vi "main_v1.2.vi"() -> ()   [LabVIEW 2012]
uses:
  SensorSettingCtl.ctl
  SensorTypes.ctl
  states.ctl
  globalVariables.vi
  <vilib>/Analysis/NI_AALPro.lvlib
panel:
  out "mean current CAN - ANA new":dbl format="%#_5g"
  out "mean currents":dbl[](array[numeric]) format="%#_5g"
  out "min dt":dbl[](array[numeric])
  out "max dt":dbl[](array[numeric])
  out "dt":dbl[][](array[numeric])
  out "end-time / s":dbl[](array[numeric])
  out "start-time / s":dbl[](array[numeric])
  out "calculated sampling rates / s":dbl[](array[numeric]) format="%^#_5e"
  out "currents zoomed 2":cluster{dbl[], dbl[]}[](graph)
  out "zoomed currents":dbl[][](array[numeric])
  out "zoomed times":dbl[][](array[numeric])
  in  "autostart":bool=TRUE
  out "raw currents":dbl[][](array[numeric])
  in  "start-indices":i32[](array[numeric])
  in  "end-indices":i32[](array[numeric])
  out "raw times":dbl[][](array[numeric])
  in  "cancel button data analysis":bool
  out "meas. time / s":dbl format="%#.1f"
  in  "max. meas. time / s":dbl=10.0
  out "measuring":bool
  out "currents raw":cluster{dbl[], dbl[]}[](graph)
  out "currents zoomed":cluster{dbl[], dbl[]}[](graph)
  in  "size of buffer":i32=1000000
  in  "Path for measuring results":path=path "C:/Users/Induelec/Desktop/test_output"
  in  "Sensor types":T1[](array[typedef])=[enum."ITL 900 (Analogue)", enum."CAB 300-C SP3 (CAN)", enum."xyz TODO (PWM)", enum."xyz TODO (LIN)", enum."xyz TODO (Analogue)"]
  in  "Sensor-enabling":T2[](array[typedef])=[{"VISA resource name"="", "use sensor"=FALSE}, {"VISA resource name"="", "use sensor"=TRUE}, {"VISA resource name"="", "use sensor"=FALSE}, {"VISA resource name"="", "use sensor"=FALSE}, {"VISA resource name"="", "use sensor"=FALSE}]
  in  "cancel button":bool
  in  "start Button":bool
  out "Error Flag":bool
  # "Measurement of Current Sensors from LEM"
  # "ANA"
  # "CAN"
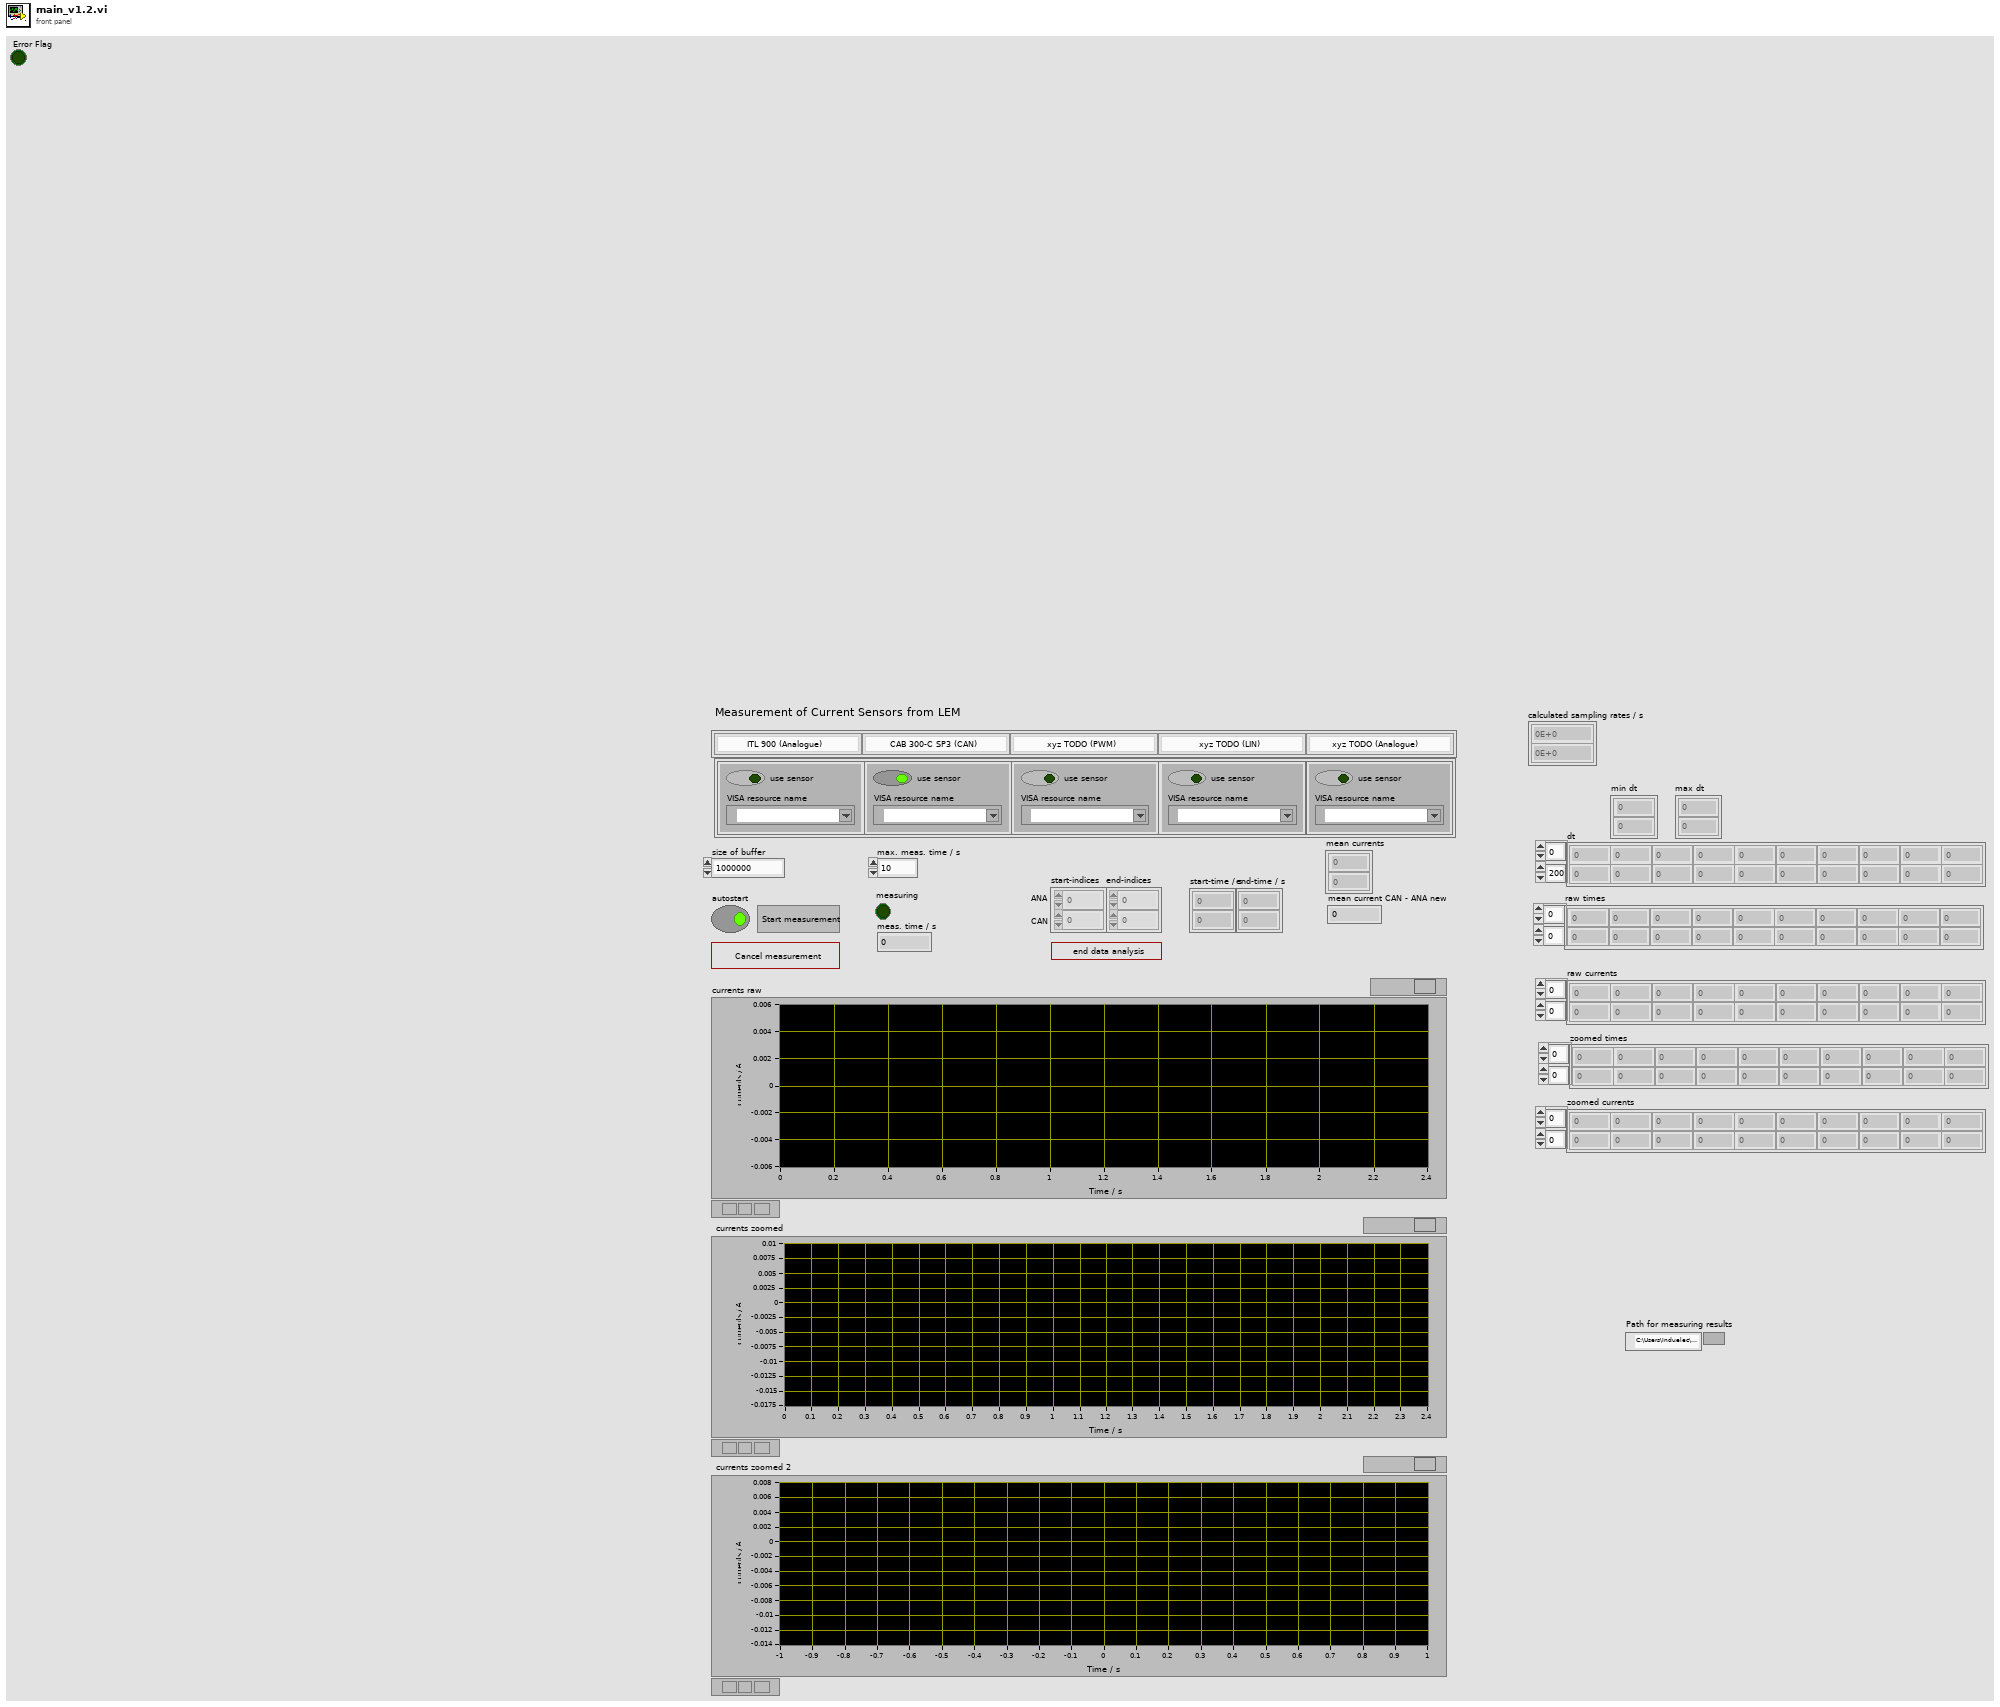
[diagram p1: front panel]
types:
  T1 = typedef "SensorTypes.ctl" = enum16{"ITL 900 (Analogue)", "CAB 300-C SP3 (CAN)", "xyz TODO (PWM)", "xyz TODO (LIN)", "xyz TODO (Analogue)"}
  T2 = typedef "SensorSettingCtl.ctl" = cluster{"VISA resource name":refnum<visa-resource-name>, "use sensor":bool}
  T3 = typedef "states.ctl" = enum16{"init", "wait for user confirm", "start sensors", "measure", "data preparation", "data analysis", "terminate"}
  T4 = typedef "Semaphore RefNum" = refnum<k1>
  T5 = typedef "TimeValue.ctl" = cluster{"Time of measurement":timestamp, "Current value":dbl}
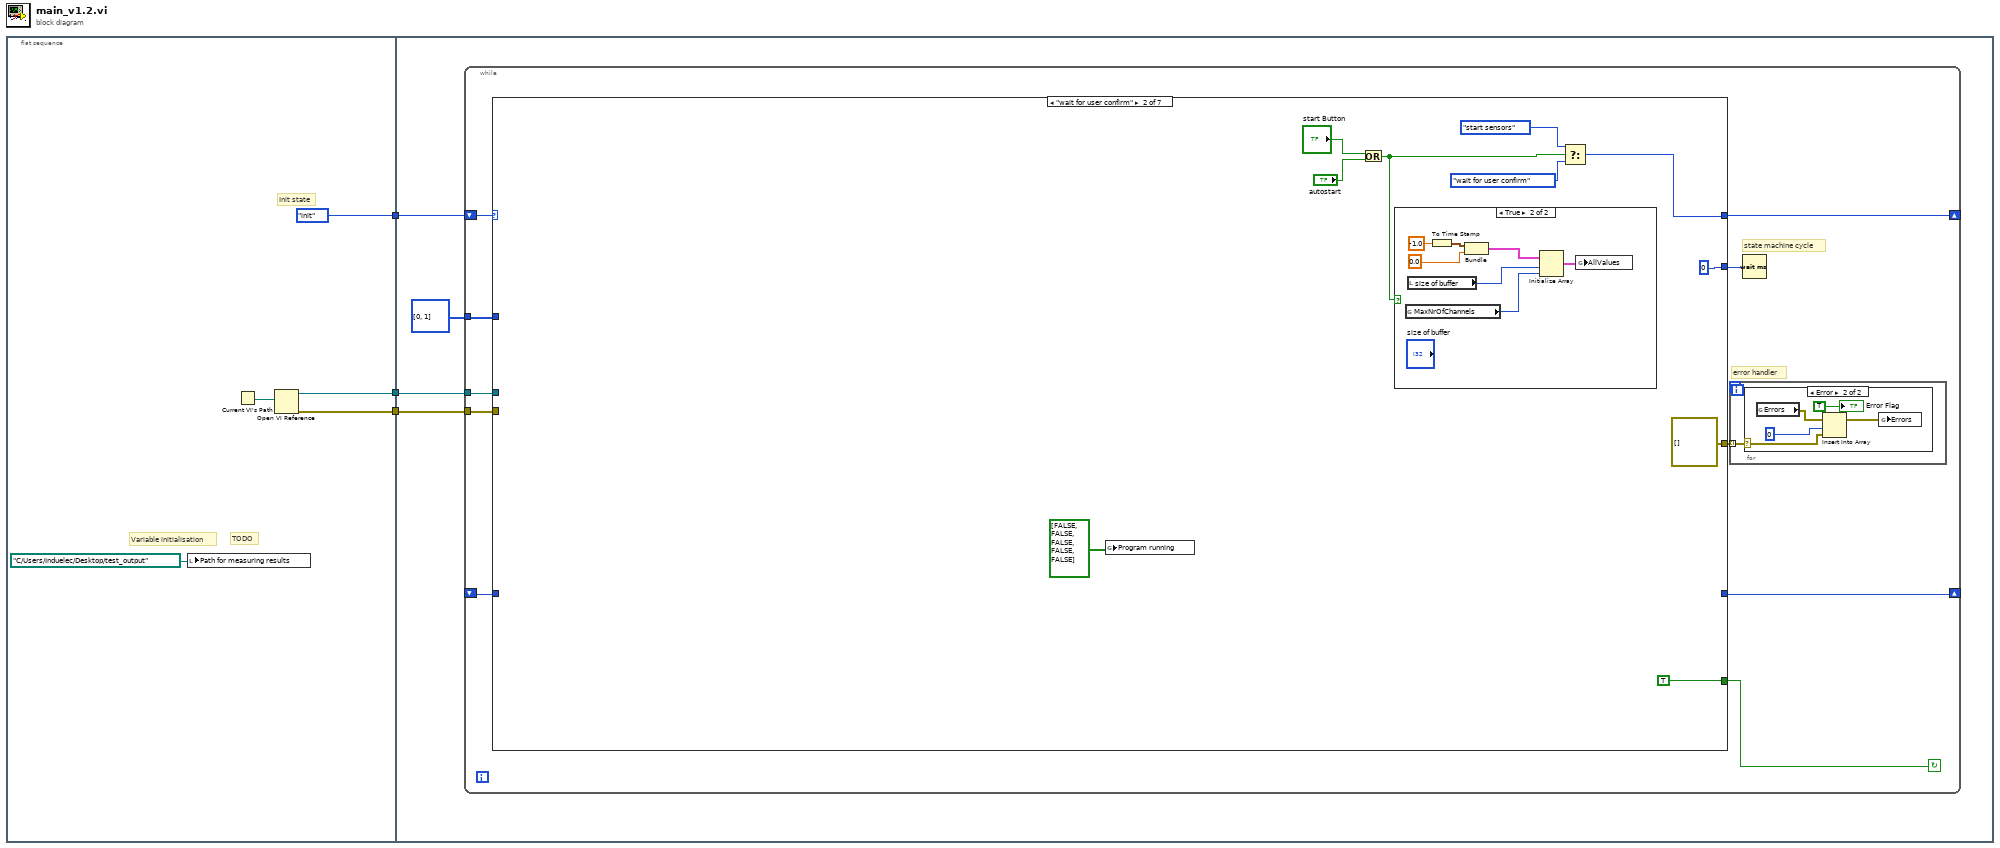
[diagram p0: block diagram]
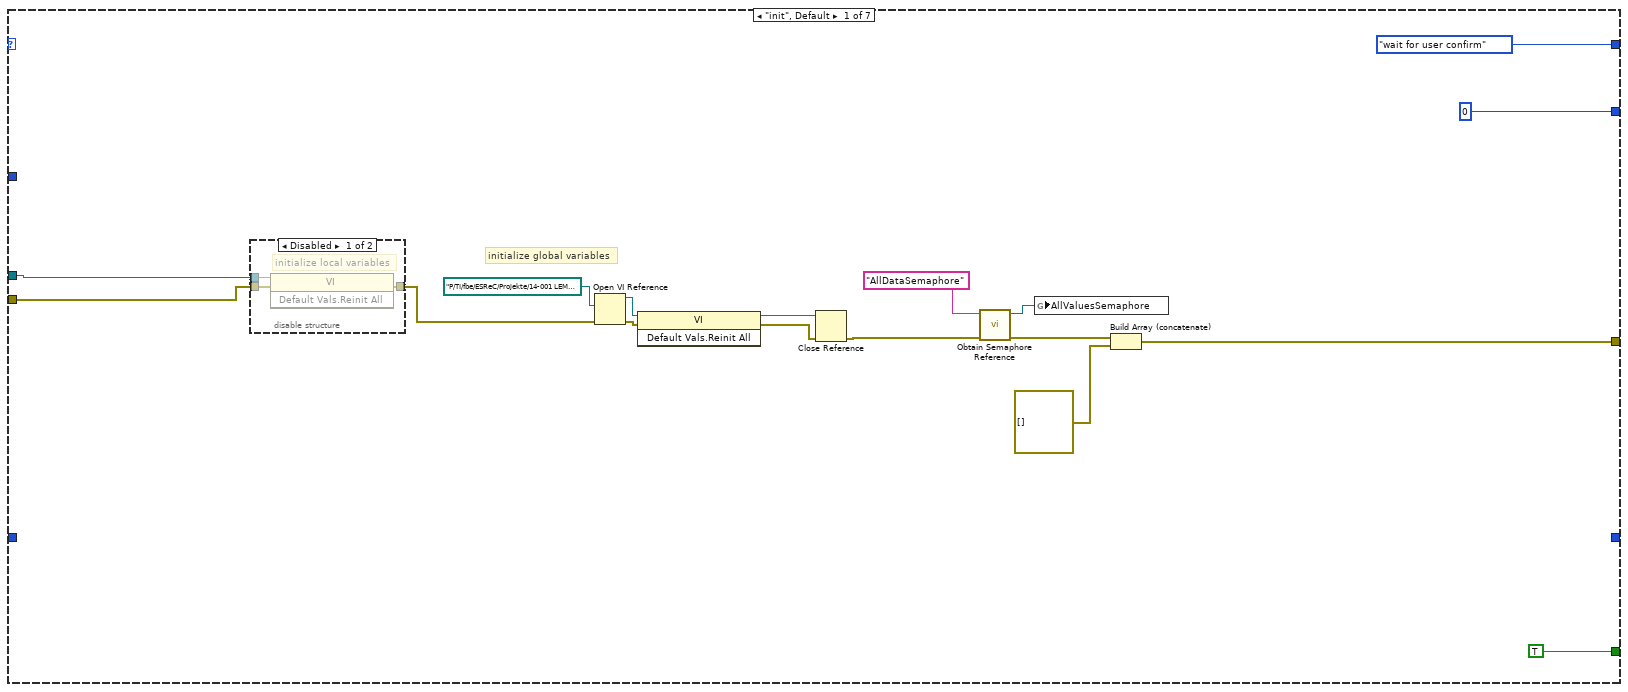
[diagram p3: hidden frame]
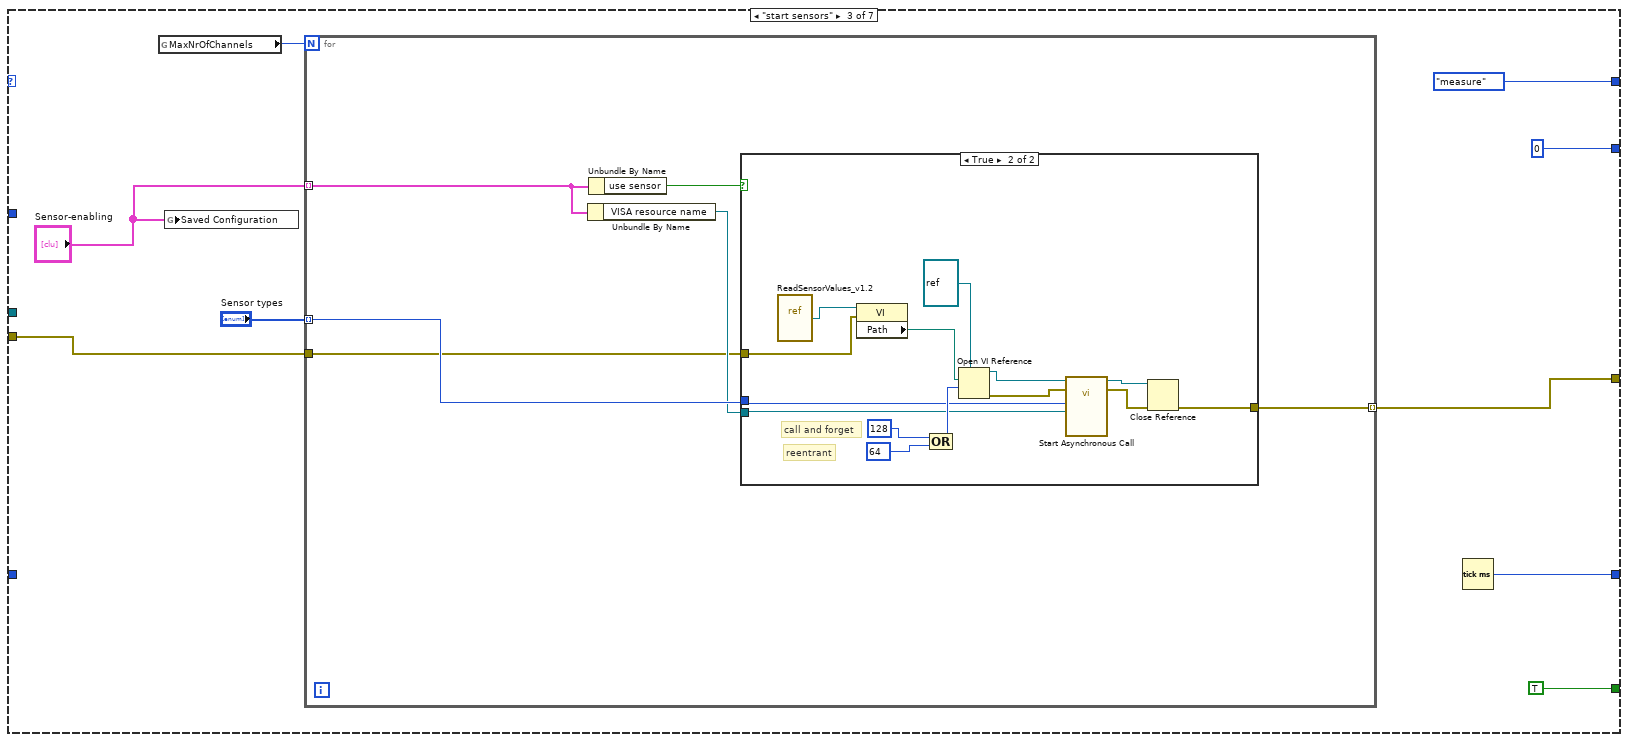
[diagram p6: hidden frame]
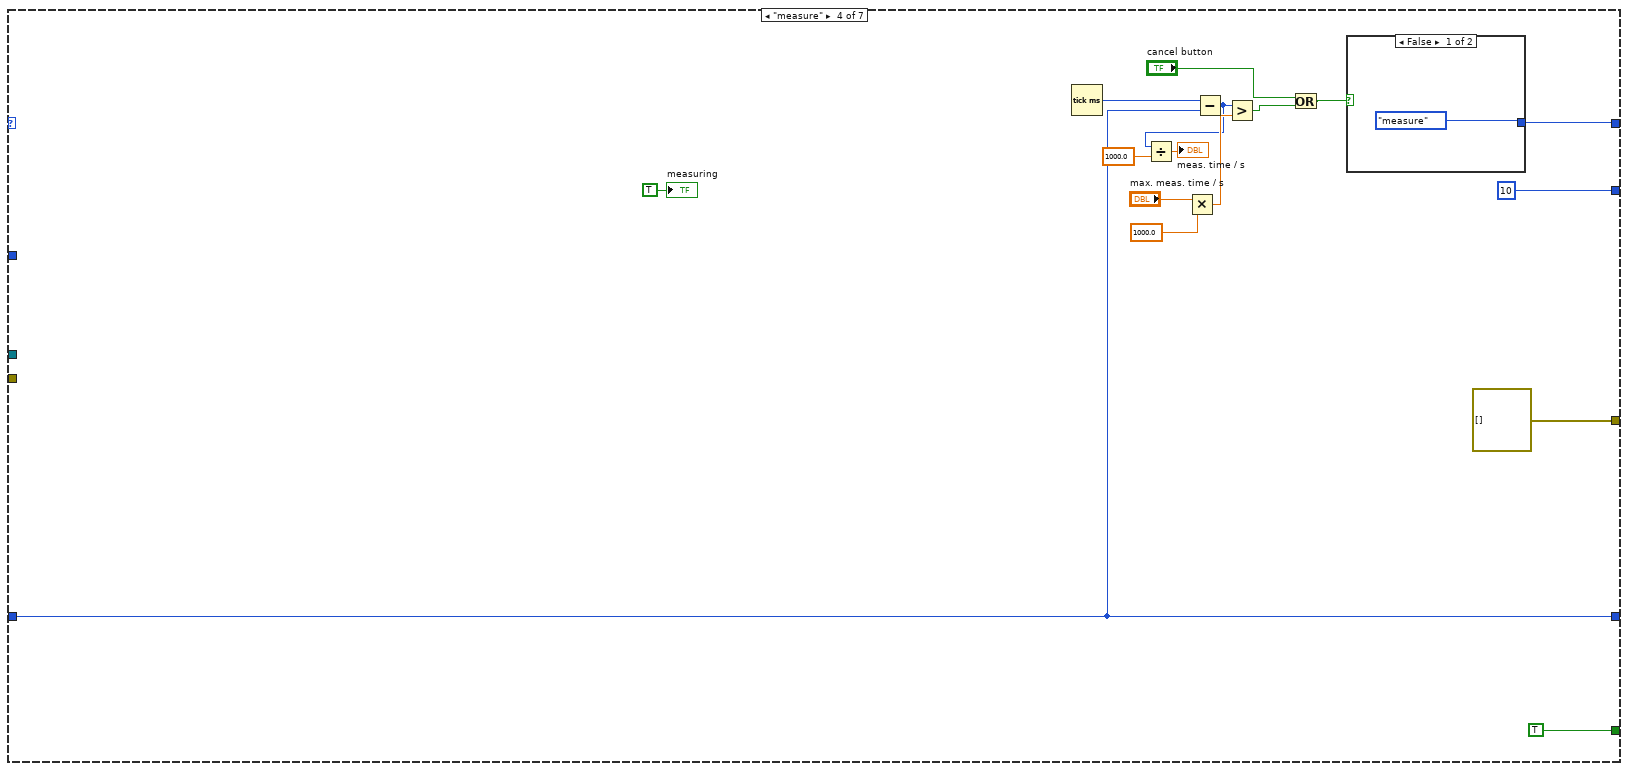
[diagram p8: hidden frame]
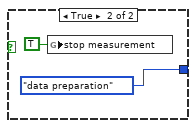
[diagram p9: hidden frame]
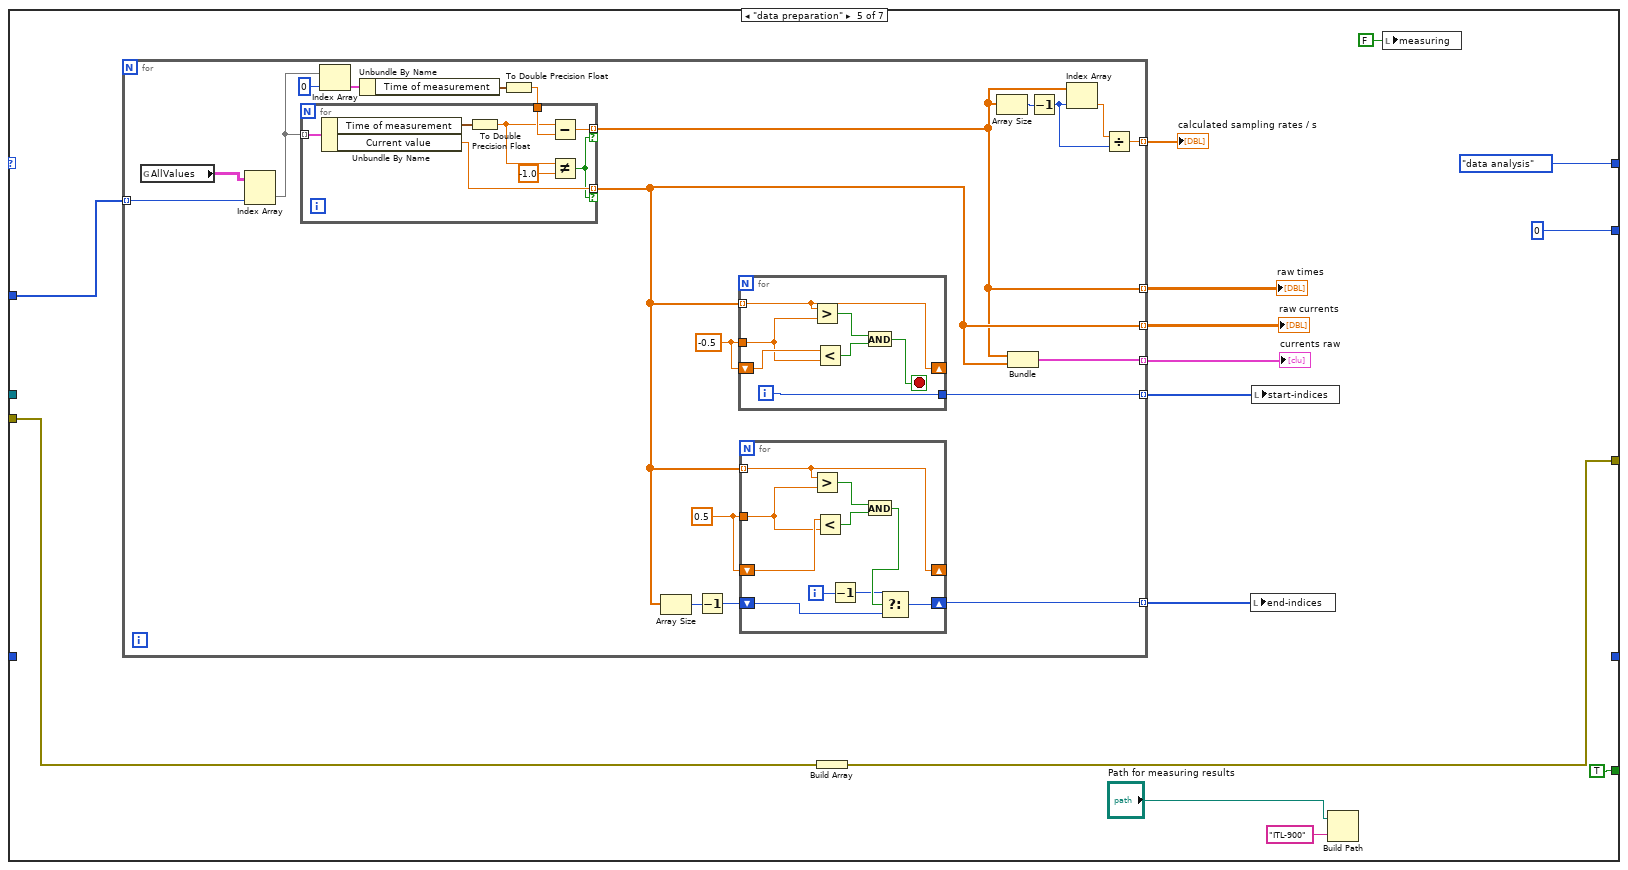
[diagram p10: hidden frame]
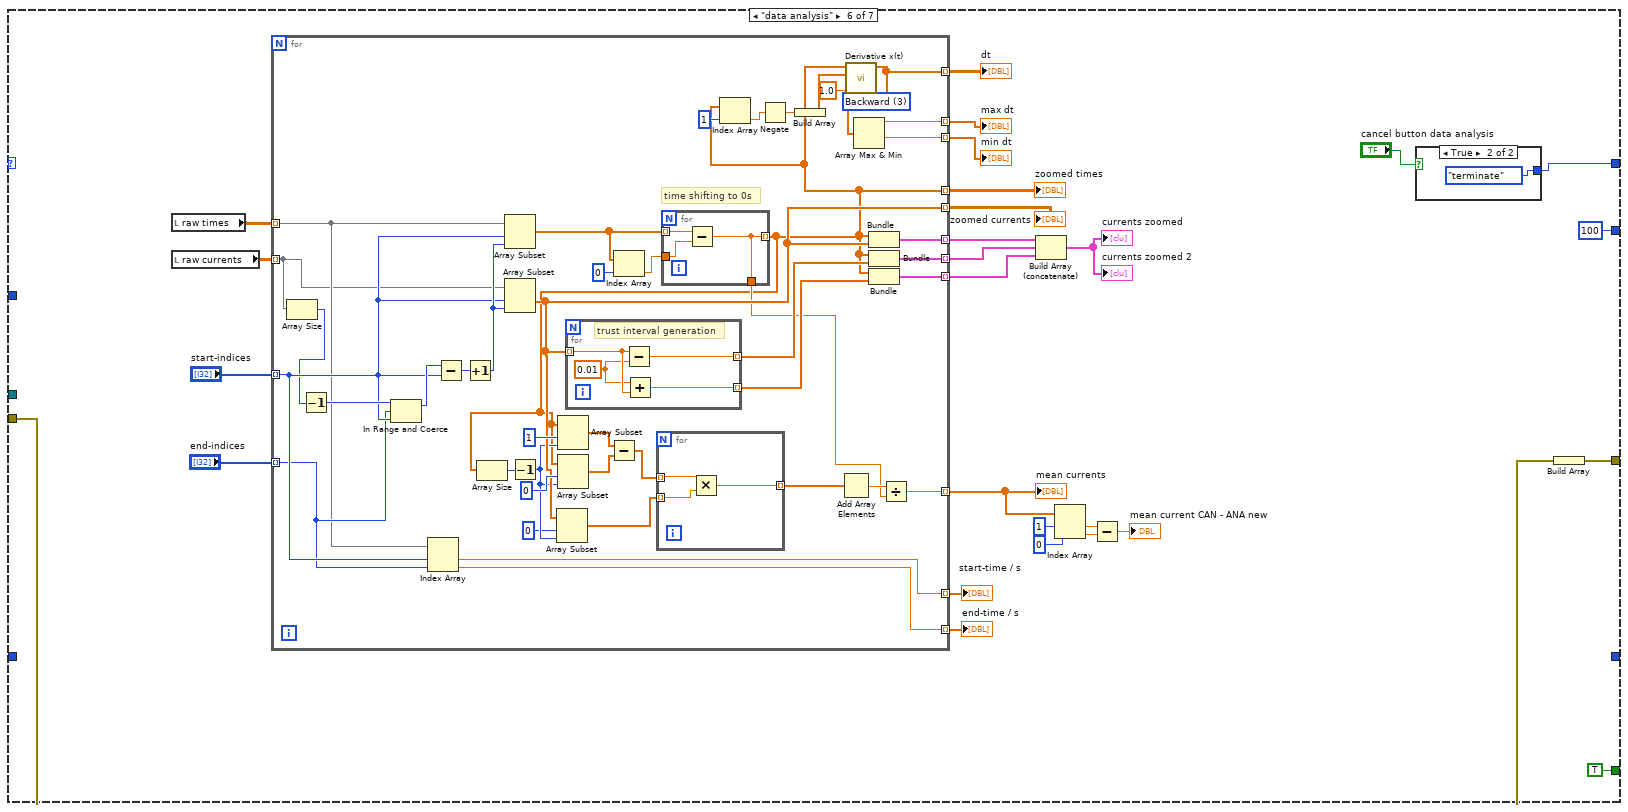
[diagram p11: hidden frame]
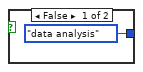
[diagram p12: hidden frame]
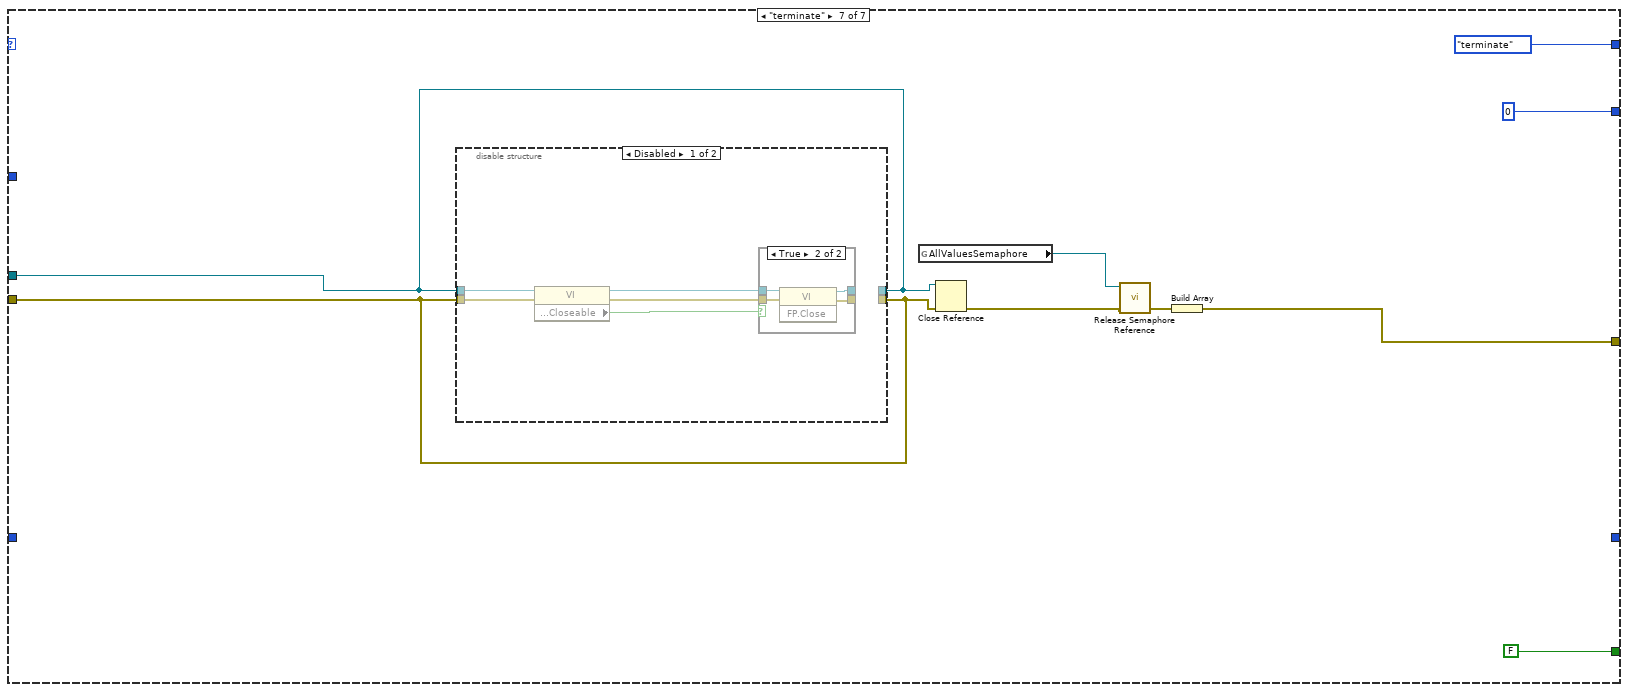
[diagram p13: hidden frame]
diagram:
  n1 = flat-sequence {
    tunnel: [states."init" ("States IEEE-488")] -> w3
    tunnel: [w8] -> w2
    tunnel: [w7] -> w1
    tunnel: w3 -> [w10]
    tunnel: w2 -> [w12]
    tunnel: w1 -> [w11]
    frame #0 {
      # "TODO"
      # "Variable initialisation"
      # "Init state"
      n2 = local write "Path for measuring results"(path "C:/Users/Induelec/Desktop/test_output" ("Path for measuring results")) -> ()
      n3 = Current VI's Path() -> (path=w6:path)
      n4 = Open VI Reference(vi path=w6) -> (vi reference=w8:refnum<vi>, error out=w7:errorcluster)  [unwired: 2 in, 3 out]
    }
    frame #1 {
      n5 = while {
        tunnel: w12 -> [w21]
        tunnel: w11 -> [w20]
        shift-right: [w17] -> _
        shift-left: w10 -> [w18]
        shift-right: [w15] -> _
        shift-left: _ -> [w14]
        tunnel: i32[] [0, 1] -> [w13]
        stop <- w16 continue-if-true
        # "error handler"
        # "state machine cycle"
        n6 = case shown="\"wait for user confirm\"" w18 {
          tunnel: [u32 0 ("milliseconds to wait") u32 0 ("milliseconds to wait") u32 0 ("milliseconds to wait") u32 10 ("milliseconds to wait") u32 0 ("milliseconds to wait") u32 100 ("milliseconds to wait") u32 0 ("milliseconds to wait")] -> w22
          tunnel: w21 -> [w42 _ _ _ _ _ w261]
          tunnel: w20 -> [w43 _ w67 _ w125 w190 w260]
          tunnel: [w44 errorcluster[] [] w72 errorcluster[] [] w126 w191 w264] -> w19
          tunnel: [states."wait for user confirm" ("States IEEE-488") w56 states."measure" ("States IEEE-488") w110 states."data analysis" ("f") w193 states."terminate" ("f")] -> w17
          tunnel: [TRUE TRUE TRUE TRUE TRUE TRUE FALSE] -> w16
          tunnel: [_ _ w66 w104 _ _ _] -> w15
          tunnel: w14 -> [_ _ _ w104 _ _ _]
          tunnel: w13 -> [_ _ _ _ w118 _ _]
          frame "init", Default {
            # "initialize global variables"
            n7 = disable-structure shown="Disabled" {
              disable-tunnel: w43 -> [w48 _]
              disable-tunnel: w42 -> [w47 _]
              disable-tunnel: [w46 _] -> w36
              frame Disabled {
                # "initialize local variables"
                n8 = invoke class="VI" method="Default Vals.Reinit All"(reference=w47, error in=w48) -> (error out=w46:errorcluster)  [unwired: 1 in, 2 out]
              }
              frame Enabled {
              }
            }
            n9 = Open VI Reference(vi path=path "P:/TI/fbe/ESReC/Projekte/14-001 LEM Current Sensor Measurements/Software/LabVIEW/Current sensor tests/globalVariables.vi", error in (no error)=w36) -> (vi reference=w37:refnum<vi>, error out=w35:errorcluster)  [unwired: 4 in]
            n10 = invoke class="VI" method="Default Vals.Reinit All"(reference=w37, error in=w35) -> (reference out=w34:refnum<vi>, error out=w33:errorcluster)  [unwired: 1 in, 1 out]
            n11 = Close Reference(reference=w34, error in (no error)=w33) -> (error out=w31:errorcluster)
            n12 = call <vilib>:"Obtain Semaphore Reference.vi"("error in (no error)"=w31, "name (unnamed)"="AllDataSemaphore") -> ("error out"=w30:errorcluster, "semaphore"=w29:T4)  [unwired: 3 in, 1 out]
            n13 = global write "globalVariables.vi" "AllValuesSemaphore"(w29) -> ()
            n14 = Build Array (concatenate)(w30, errorcluster[] [] ("array")) -> (w44:errorcluster[])
          }
          frame "wait for user confirm" {
            n15 = global write "globalVariables.vi" "Program running"(bool[] [FALSE, FALSE, FALSE, FALSE, FALSE] ("Program running")) -> ()
            n16 = Or(x="start Button", y="autostart") -> (x .or. y?=w51:bool)
            n17 = case shown="True" w51 {
              frame False {
              }
              frame True {
                n18 = global read "globalVariables.vi" "MaxNrOfChannels"() -> (w65:i32)
                n19 = local read "size of buffer"() -> (w63:i32)
                n20 = To Time Stamp(1:-1.0 ("number")) -> (0:w61:timestamp)
                n21 = Bundle(w61, 0.0) -> (w59:cluster{timestamp, dbl})  [unwired: 1 in]
                n22 = Initialize Array(w59, w63, w65) -> (w64:cluster{timestamp, dbl}[][])
                n23 = global write "globalVariables.vi" "AllValues"(w64) -> ()
              }
            }
            n24 = Select(t=states."start sensors" ("States IEEE-488"), s=w51, f=states."wait for user confirm" ("States IEEE-488")) -> (s? t:f=w56:T3)
          }
          frame "start sensors" {
            n25 = global read "globalVariables.vi" "MaxNrOfChannels"() -> (w69:i32)
            n26 = global write "globalVariables.vi" "Saved Configuration"("Sensor-enabling") -> ()
            n27 = for {
              N: w69 -> [_]
              tunnel: "Sensor-enabling" -> [w79] mode=indexing
              tunnel: [w78] -> w72 mode=indexing
              tunnel: "Sensor types" -> [w77] mode=indexing
              tunnel: w67 -> [w75]
              n28 = Unbundle By Name(w79) -> ("VISA resource name"=w76:refnum<visa-resource-name>)
              n29 = Unbundle By Name(w79) -> ("use sensor"=w80:bool)
              n30 = case shown="True" w80 {
                tunnel: [w81 w93] -> w78
                tunnel: w77 -> [_ w86]
                tunnel: w76 -> [_ w85]
                tunnel: w75 -> [w81 w87]
                frame False {
                }
                frame True {
                  # "reentrant"
                  # "call and forget"
                  n31 = vi-ref "ReadSensorValues_v1.2.vi"() -> (w83:refnum<vi>)
                  n32 = property class="VI"(reference=w83, error in=w87) -> ("Path"=w95:path)  [unwired: 2 out]
                  n33 = Compound Arithmetic op=OR(128 ("options"), 64 ("value")) -> (w92:i32)
                  n34 = Open VI Reference(type specifier VI Refnum (for type only)=refnum<vi> refnum, vi path=w95, options=w92) -> (vi reference=w82:refnum<vi>, error out=w90:errorcluster)  [unwired: 3 in]
                  n35 = call-by-ref "Start Asynchronous Call"(reference=w82, error in=w90, "VISA resource name"=w85, "Sensor type"=w86) -> (reference out=w89:refnum<vi>, error out=w88:errorcluster)  [unwired: 2 in]
                  n36 = Close Reference(reference=w89, error in (no error)=w88) -> (error out=w93:errorcluster)
                }
              }
            }
            n37 = Tick Count (ms)() -> (millisecond timer value=w66:u32)
          }
          frame "measure" {
            n38 = Tick Count (ms)() -> (millisecond timer value=w98:u32)
            n39 = Multiply(x="max. meas. time / s", y=1000.0) -> (x*y=w101:dbl)
            n40 = Subtract(x=w98, y=w104) -> (x-y=w96:u32)
            n41 = Divide(x=w96, y=1000.0) -> (x/y=→"meas. time / s":dbl)
            n42 = Greater?(x=w96, y=w101) -> (0:w105:bool)
            n43 = Or(x="cancel button", y=w105) -> (x .or. y?=w107:bool)
            n44 = case shown="False" w107 {
              tunnel: [states."measure" ("f") states."data preparation" ("States IEEE-488")] -> w110
              frame False {
              }
              frame True {
                n45 = global write "globalVariables.vi" "stop measurement"(TRUE ("stop measurement")) -> ()
              }
            }
            "measuring" <- TRUE ("measuring")
          }
          frame "data preparation" {
            n46 = for {
              tunnel: w118 -> [w144] mode=indexing
              tunnel: [w132] -> w116 mode=indexing
              tunnel: [w136] -> w120 mode=indexing
              tunnel: [w138] -> w121 mode=indexing
              tunnel: [w137] -> w122 mode=indexing
              tunnel: [w135] -> w119 mode=indexing
              tunnel: [w134] -> w115 mode=indexing
              w139 = -0.5
              w140 = 0.5
              n47 = global read "globalVariables.vi" "AllValues"() -> (w149:T5[][])
              n48 = Index Array(array=w149, index (col)=w144) -> (element=w143:T5[])  [unwired: 1 in]
              n49 = Index Array(array=w143, index=0) -> (element=w147:T5)
              n50 = Unbundle By Name(w147) -> ("Time of measurement"=w146:timestamp)
              n51 = To Double Precision Float(number=w146) -> (double precision float=w145:dbl)
              n52 = for {
                tunnel: w143 -> [w174] mode=indexing
                tunnel: [w167] -> w132 mode=indexing if=w168
                tunnel: [w172] -> w136 mode=indexing if=w168
                tunnel: w145 -> [w171]
                n53 = Unbundle By Name(w174) -> ("Time of measurement"=w173:timestamp, "Current value"=w172:dbl)
                n54 = To Double Precision Float(number=w173) -> (double precision float=w169:dbl)
                n55 = Subtract(x=w169, y=w171) -> (x-y=w167:dbl)
                n56 = Not Equal?(x=w169, y=-1.0) -> (x != y?=w168:bool)
              }
              n57 = Array Size(array=w136) -> (size(s)=w142:i32)
              n58 = Decrement(x=w142) -> (x-1=w141:i32)
              n59 = for {
                tunnel: w136 -> [w162] mode=indexing
                tunnel: [w166] -> w137
                shift-right: [w162] -> _
                shift-left: w139 -> [w161]
                tunnel: w139 -> [w160]
                i -> [w166]
                stop <- w164 stop-if-true
                n60 = Greater?(x=w162, y=w160) -> (0:w163:bool)
                n61 = Less?(x=w161, y=w160) -> (x < y?=w165:bool)
                n62 = And(x=w163, y=w165) -> (x .and. y?=w164:bool)
              }
              n63 = for {
                tunnel: w136 -> [w154] mode=indexing
                shift-right: [w159] -> w138
                shift-left: w141 -> [w158]
                shift-right: [w154] -> _
                shift-left: w140 -> [w153]
                tunnel: w140 -> [w152]
                i -> [w151]
                n64 = Greater?(x=w154, y=w152) -> (0:w157:bool)
                n65 = Less?(x=w153, y=w152) -> (x < y?=w156:bool)
                n66 = Decrement(x=w151) -> (x-1=w150:i32)
                n67 = And(x=w157, y=w156) -> (x .and. y?=w155:bool)
                n68 = Select(t=w150, s=w155, f=w158) -> (s? t:f=w159:i32)
              }
              n69 = Array Size(array=w132) -> (size(s)=w131:i32)
              n70 = Bundle(w132, w136) -> (w135:cluster{dbl[], dbl[]})  [unwired: 1 in]
              n71 = Decrement(x=w131) -> (x-1=w130:i32)
              n72 = Index Array(array=w132, index=w130) -> (element=w133:dbl)
              n73 = Divide(x=w133, y=w130) -> (x/y=w134:dbl)
            }
            "raw times" <- w116
            "currents raw" <- w119
            "raw currents" <- w120
            "calculated sampling rates / s" <- w115
            n74 = Build Array(w125) -> (w126:errorcluster[])
            n75 = local write "end-indices"(w121) -> ()
            n76 = local write "start-indices"(w122) -> ()
            n77 = Build Path(base path="Path for measuring results", name or relative path="ITL-900") -> ()  [unwired: 1 out]
            n78 = local write "measuring"(FALSE ("measuring")) -> ()
          }
          frame "data analysis" {
            n79 = local read "raw times"() -> (w199:dbl[][])
            n80 = local read "raw currents"() -> (w198:dbl[][])
            n81 = for {
              tunnel: "start-indices" -> [w210] mode=indexing
              tunnel: "end-indices" -> [w209] mode=indexing
              tunnel: w199 -> [w206] mode=indexing
              tunnel: w198 -> [w205] mode=indexing
              tunnel: [w243] -> w197 mode=indexing
              tunnel: [w242] -> w196 mode=indexing
              tunnel: [w241] -> w195 mode=indexing
              tunnel: [w211] -> w184 mode=indexing
              tunnel: [w220] -> w188 mode=indexing
              tunnel: [w208] -> w186 mode=indexing
              tunnel: [w207] -> w185 mode=indexing
              tunnel: [w233] -> w183 mode=indexing
              tunnel: [w232] -> w182 mode=indexing
              tunnel: [w227] -> w181 mode=indexing
              tunnel: [w213] -> w175 mode=indexing
              w234 = u16 3 items=["2nd Order Central", "4th Order Central", "Forward", "Backward"] ("method")
              # "time shifting to 0s"
              n82 = Array Size(array=w205) -> (size(s)=w204:i32)
              n83 = Decrement(x=w204) -> (x-1=w246:i32)
              n84 = In Range and Coerce(upper limit=w246, x=w209, lower limit=w210) -> (coerced(x)=w240:i32)  [unwired: 1 out]
              n85 = Index Array(array=w206, index #1=w210, index #2=w209) -> (element #1=w208:dbl, element #2=w207:dbl)
              n86 = Subtract(x=w240, y=w210) -> (x-y=w239:i32)
              n87 = Increment(x=w239) -> (x+1=w238:i32)
              n88 = Array Subset(array=w206, index=w210, length=w238) -> (w224:dbl[])
              n89 = Array Subset(array=w205, index=w210, length=w238) -> (w220:dbl[])
              n90 = for {
                tunnel: w220 -> [w256] mode=indexing
                tunnel: [w254] -> w236 mode=indexing
                tunnel: [w253] -> w245 mode=indexing
                w255 = 0.01
                # "trust interval generation"
                n91 = Subtract(x=w256, y=w255) -> (x-y=w254:dbl)
                n92 = Add(x=w255, y=w256) -> (x+y=w253:dbl)
              }
              n93 = Index Array(array=w224, index=0) -> (element=w237:dbl)
              n94 = for {
                tunnel: w237 -> [w251]
                tunnel: w224 -> [w252] mode=indexing
                tunnel: [w250] -> w211 mode=indexing
                tunnel: [w250] -> w212
                n95 = Subtract(x=w252, y=w251) -> (x-y=w250:dbl)
              }
              n96 = Array Size(array=w211) -> (size(s)=w225:i32)
              n97 = Decrement(x=w225) -> (x-1=w219:i32)
              n98 = Array Subset(array=w220, index=0, length=w219) -> (w216:dbl[])
              n99 = Array Subset(array=w211, index=1, length=w219) -> (w222:dbl[])
              n100 = Array Subset(array=w211, index=0, length=w219) -> (w221:dbl[])
              n101 = Subtract(x=w222, y=w221) -> (x-y=w217:dbl[])
              n102 = for {
                tunnel: w217 -> [w249] mode=indexing
                tunnel: w216 -> [w248] mode=indexing
                tunnel: [w247] -> w215 mode=indexing
                n103 = Multiply(x=w249, y=w248) -> (x*y=w247:dbl)
              }
              n104 = Index Array(array=w211, index=1) -> (element=w230:dbl)
              n105 = Negate(x=w230) -> (-x=w229:dbl)
              n106 = Build Array(w229) -> (w228:dbl[])
              n107 = Add Array Elements(numeric array=w215) -> (sum=w214:dbl)
              n108 = call <vilib>:"Derivative x(t).vi"("method"=w234, "dt"=1.0, "Initial Condition"=w228, "X"=w211) -> ("dX/dt"=w227:dbl[])  [unwired: 6 in, 1 out]
              n109 = Array Max & Min(array=w227) -> (max value=w233:dbl, min value=w232:dbl)  [unwired: 2 out]
              n110 = Bundle(w211, w220) -> (w243:cluster{dbl[], dbl[]})  [unwired: 1 in]
              n111 = Bundle(w211, w236) -> (w242:cluster{dbl[], dbl[]})  [unwired: 1 in]
              n112 = Bundle(w211, w245) -> (w241:cluster{dbl[], dbl[]})  [unwired: 1 in]
              n113 = Divide(x=w214, y=w212) -> (x/y=w213:dbl)
            }
            "zoomed times" <- w184
            "zoomed currents" <- w188
            "start-time / s" <- w186
            "end-time / s" <- w185
            "dt" <- w181
            "max dt" <- w183
            "min dt" <- w182
            "mean currents" <- w175
            n114 = Build Array (concatenate)(w197, w196, w195) -> (→"currents zoomed" →"currents zoomed 2":cluster{dbl[], dbl[]}[])
            n115 = Index Array(array=w175, index #1=1 ("index"), index #2=0 ("index")) -> (element #1=w177:dbl, element #2=w178:dbl)
            n116 = Subtract(x=w177, y=w178) -> (x-y=→"mean current CAN - ANA new":dbl)
            n117 = case shown="True" "cancel button data analysis" {
              tunnel: [states."data analysis" ("f") states."terminate" ("f")] -> w193
              frame False {
              }
              frame True {
              }
            }
            n118 = Build Array(w190) -> (w191:errorcluster[])
          }
          frame "terminate" {
            n119 = disable-structure shown="Disabled" {
              disable-tunnel: w260 -> [w267 _]
              disable-tunnel: w261 -> [w266 _]
              disable-tunnel: w261 -> [_ _]
              disable-tunnel: w260 -> [_ _]
              frame Disabled {
                n120 = property class="VI"(reference=w266, error in=w267) -> (reference out=w269:refnum<vi>, error out=w268:errorcluster, "Front Panel.Closeable"=w270:bool)
                n121 = case shown="True" w270 {
                  tunnel: w269 -> [w272 w276]
                  tunnel: [w272 w275] -> _
                  tunnel: w268 -> [w271 w274]
                  tunnel: [w271 w273] -> _
                  frame False {
                  }
                  frame True {
                    n122 = invoke class="VI" method="FP.Close"(reference=w276, error in=w274) -> (reference out=w275:refnum<vi>, error out=w273:errorcluster)  [unwired: 1 in, 1 out]
                  }
                }
              }
              frame Enabled {
              }
            }
            n123 = global read "globalVariables.vi" "AllValuesSemaphore"() -> (w257:T4)
            n124 = Close Reference(reference=w261, error in (no error)=w260) -> (error out=w259:errorcluster)
            n125 = call <vilib>:"Release Semaphore Reference.vi"("error in (no error)"=w259, "semaphore"=w257) -> ("error out"=w258:errorcluster)  [unwired: 8 in, 1 out]
            n126 = Build Array(w258) -> (w264:errorcluster[])
          }
        }
        n127 = for {
          tunnel: w19 -> [w23] mode=indexing
          n128 = case shown="Error" w23 {
            selector: w23 -> [_ w27]
            frame No Error {
            }
            frame Error {
              n129 = global read "globalVariables.vi" "Errors"() -> (w25:errorcluster[])
              n130 = Insert Into Array(array=w25, index=0, new element=w27) -> (w24:errorcluster[])
              n131 = global write "globalVariables.vi" "Errors"(w24) -> ()
              "Error Flag" <- TRUE ("Error Flag")
            }
          }
        }
        n132 = Wait (ms)(milliseconds to wait=w22) -> ()  [unwired: 1 out]
      }
    }
  }
